vi "array demo.vi"() -> ()   [LabVIEW 2011]
panel:
  in  "stop":bool
  in  "add to array":bool
  in  "enter number":dbl format="%.6g"
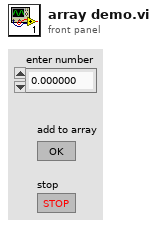
[diagram p1: front panel]
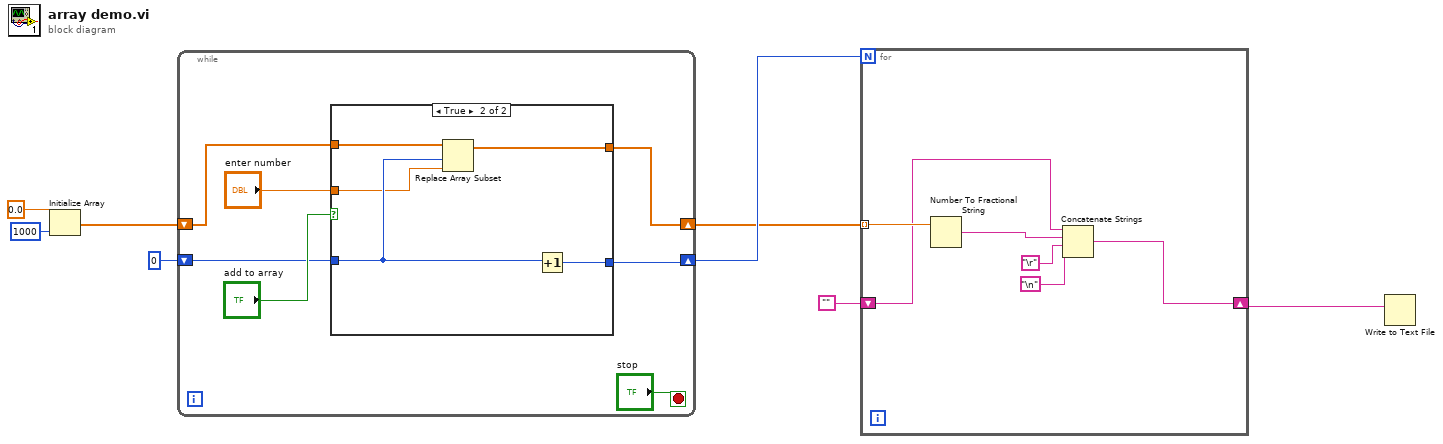
[diagram p0: block diagram]
diagram:
  n1 = Initialize Array(0.0 ("element"), 1000 ("dimension size")) -> (w6:dbl[])
  n2 = while {
    shift-right: [w9] -> w3
    shift-left: w6 -> [w12]
    shift-right: [w11] -> w4
    shift-left: 0 -> [w10]
    stop <- "stop" stop-if-true
    n3 = case shown="True" "add to array" {
      tunnel: "enter number" -> [_ w19]
      tunnel: w12 -> [w16 w22]
      tunnel: [w17 w21] -> w11
      tunnel: w10 -> [w17 w20]
      tunnel: [w16 w18] -> w9
      frame False {
      }
      frame True {
        n4 = Replace Array Subset(array=w22, new element=w19, index=w20) -> (w18:dbl[])
        n5 = Increment(x=w20) -> (x+1=w21:i32)
      }
    }
  }
  n6 = for {
    N: w4 -> [_]
    tunnel: w3 -> [w28] mode=indexing
    shift-right: [w23] -> w1
    shift-left: "" -> [w27]
    n7 = Number To Fractional String(number=w28) -> (F-format string=w26:string)  [unwired: 3 in]
    n8 = Concatenate Strings(w27, w26, "\r", "\n") -> (w23:string)
  }
  n9 = Write to Text File(text=w1) -> ()  [unwired: 3 in, 3 out]
